vi "WriteValByNmVariant.vi"(7 "Ctrl Name":string, 8 "error in":errorcluster caption="entrée d'erreur", 9 "Valeur":variant, 10 "CtrlRef":refnum<vi>[](array[refnum]), 11 "ControlsNames":string[](array[string])) -> (0 "error out":errorcluster caption="sortie d'erreur", 3 "référence en sortie":refnum<vi>)   [LabVIEW 2019]
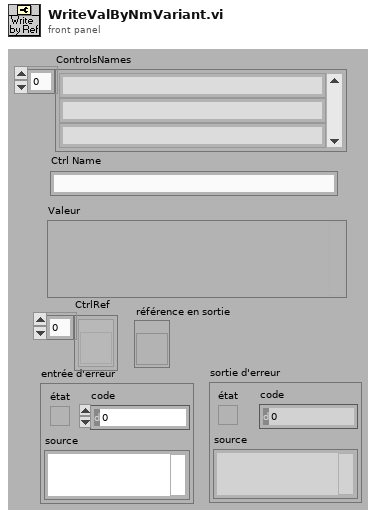
[diagram p1: front panel]
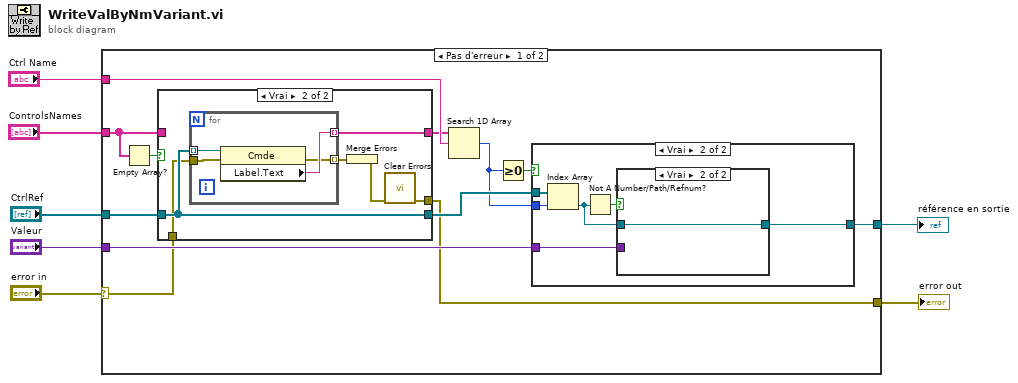
[diagram p0: block diagram]
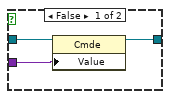
[diagram p4: hidden frame]
diagram:
  n1 = case shown="Pas d'erreur" "error in" {
    selector: "error in" -> [w9 w43]
    tunnel: "Valeur" -> [w19 _]
    tunnel: [w8 w43] -> w5
    tunnel: "ControlsNames" -> [w10 _]
    tunnel: "Ctrl Name" -> [w13 _]
    tunnel: "CtrlRef" -> [w14 _]
    tunnel: [w17 _] -> w1
    frame No Error {
      n2 = Empty Array?(array=w10) -> (empty?=w16:bool)
      n3 = case shown="Vrai" w16 {
        tunnel: [w22 w28] -> w15
        tunnel: w14 -> [w22 w28]
        tunnel: [w21 w27] -> w11
        tunnel: w10 -> [w21 _]
        tunnel: w9 -> [w20 w26]
        tunnel: [w20 w23] -> w8
        frame False {
        }
        frame True {
          n4 = for {
            tunnel: w28 -> [w32] mode=indexing
            tunnel: [w31] -> w27 mode=indexing
            tunnel: w26 -> [w30]
            tunnel: [w29] -> w25 mode=indexing
            n5 = property class="Cmde"(reference=w32, error in=w30) -> (error out=w29:errorcluster, "Label.Text"=w31:string)  [unwired: 1 out]
          }
          n6 = Merge Errors(w25) -> (w24:errorcluster)
          n7 = call <vilib>:"Clear Errors.vi"("error in (no error)"=w24) -> ("error out"=w23:errorcluster)  [unwired: 5 in, 1 out]
        }
      }
      n8 = Search 1D Array(1D array=w11, element=w13) -> (index of element=w12:i32)  [unwired: 1 in]
      n9 = Greater Or Equal To 0?(x=w12) -> (x >= 0?=w18:bool)
      n10 = case shown="Vrai" w18 {
        tunnel: w19 -> [_ w37]
        tunnel: w15 -> [_ w36]
        tunnel: w12 -> [_ w35]
        tunnel: [_ w33] -> w17
        frame False {
        }
        frame True {
          n11 = Index Array(array=w36, index=w35) -> (element=w34:refnum<vi>)
          n12 = Not A Number/Path/Refnum?(number/path/refnum=w34) -> (NaN/Path/Refnum?=w38:bool)
          n13 = case shown="Vrai" w38 {
            tunnel: w34 -> [w41 w42]
            tunnel: w37 -> [w40 _]
            tunnel: [w39 w42] -> w33
            frame False {
              n14 = property class="Cmde"(reference=w41, "Value"=w40) -> (reference out=w39:refnum<vi>)  [unwired: 1 in, 1 out]
            }
            frame True {
            }
          }
        }
      }
    }
    frame Error {
    }
  }
  "error out" <- w5
  "référence en sortie" <- w1
